vi "Main UI.vi"() -> ()   [LabVIEW 2015, in "Application.lvclass"]
uses:
  Application.lvclass
  EXECUTION_UI_STATE_TYPEDEF.ctl
  Project.lvclass
panel:
  in  "StopBtn":bool
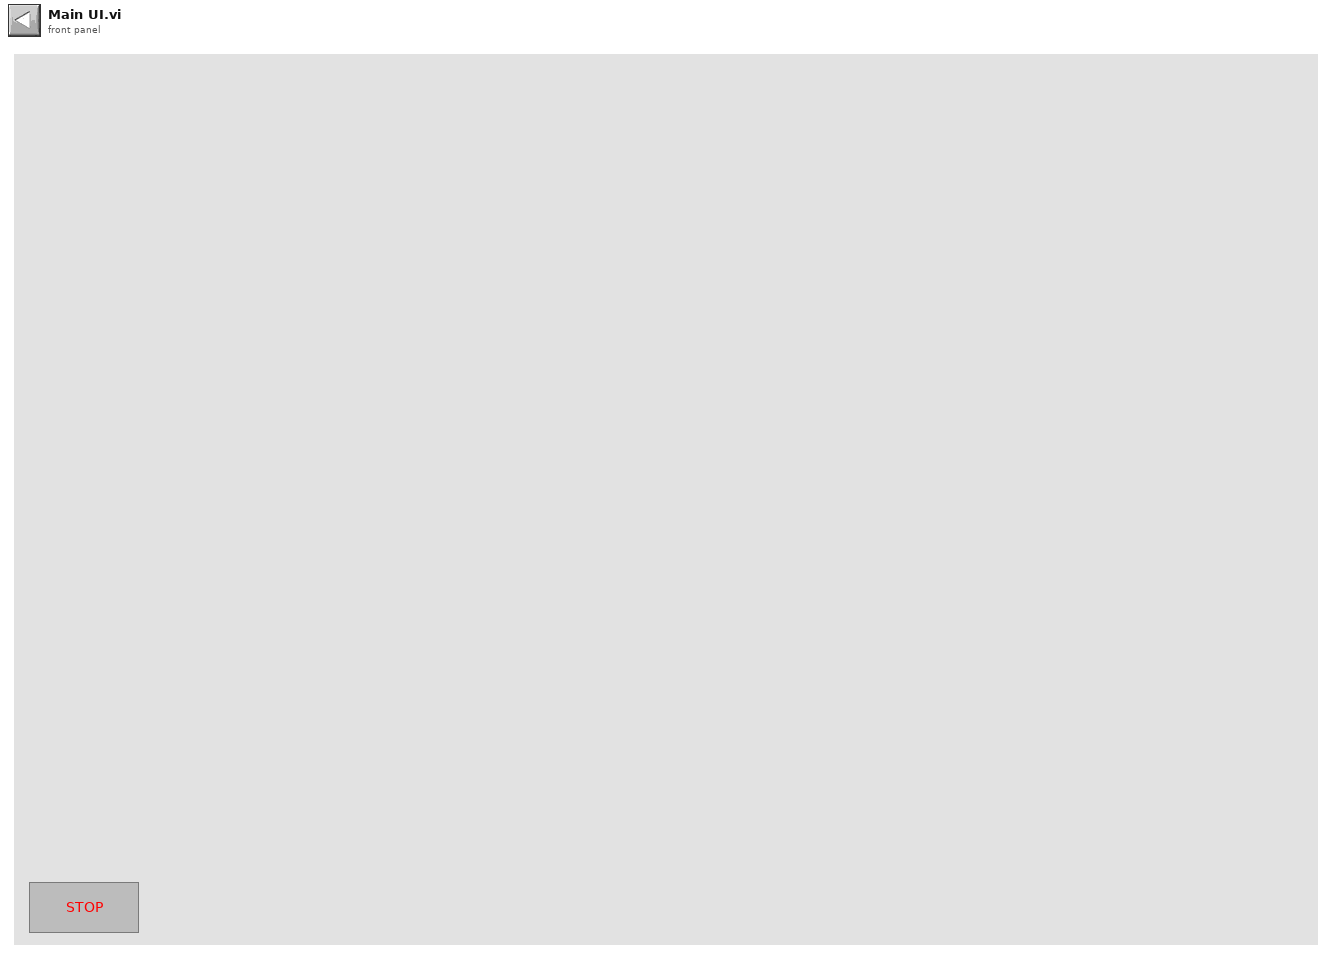
[diagram p1: front panel]
types:
  T1 = typedef "Application.lvclass/EXECUTION_UI_STATE_TYPEDEF.ctl" = enum16{"EXIT", "UI_LOOP", "LOAD_PROJ", "LOG_VIEWER", "PLUGIN_OPTIONS", "APP_OPTIONS", "ABOUT_TESTLITE"}
  T2 = enum32{"Invalid", "Standard", "Closed", "Hidden", "Minimized", "Maximized"}
  T3 = enum32{"invalid app kind", "Development System", "Run Time System", "Student Edition", "Embedded LabVIEW", "Evaluation", "Custom"}
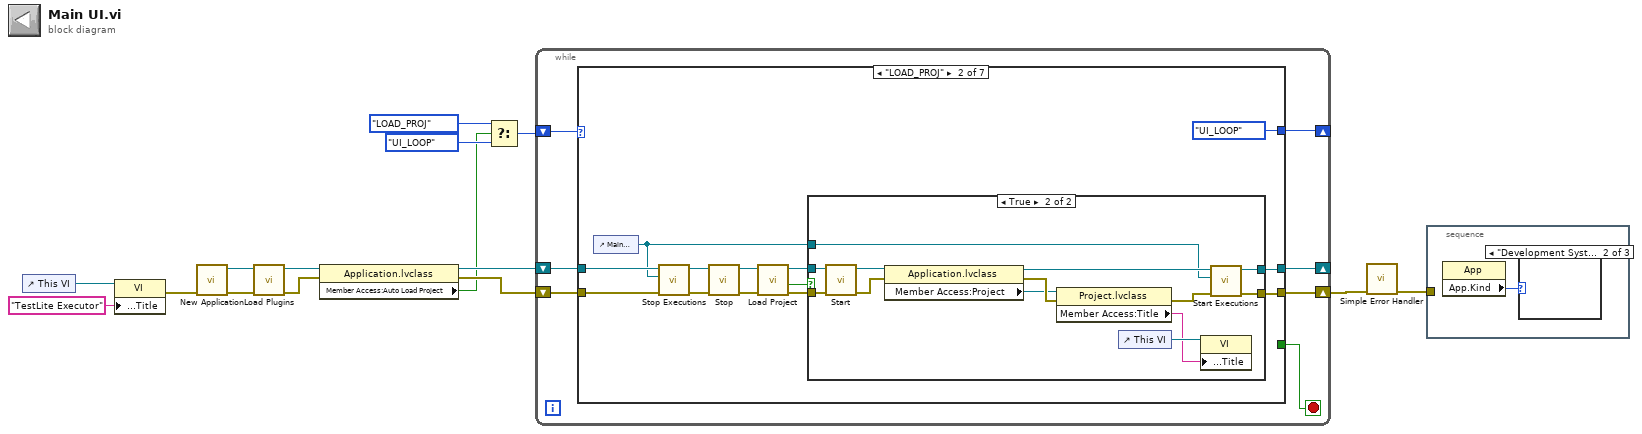
[diagram p0: block diagram]
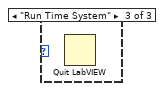
[diagram p3: hidden frame]
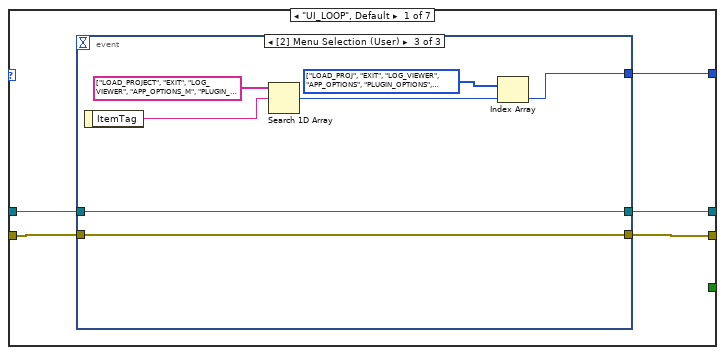
[diagram p4: hidden frame]
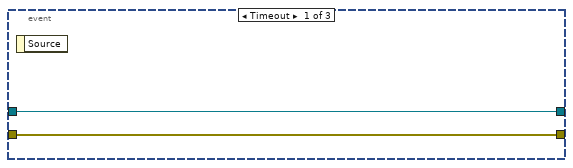
[diagram p5: hidden frame]
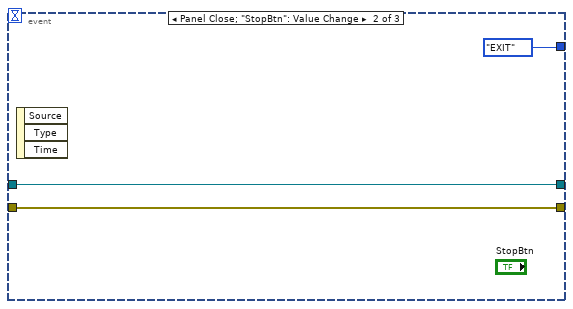
[diagram p6: hidden frame]
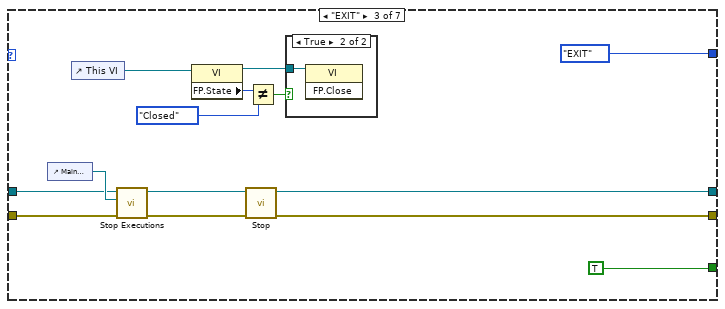
[diagram p8: hidden frame]
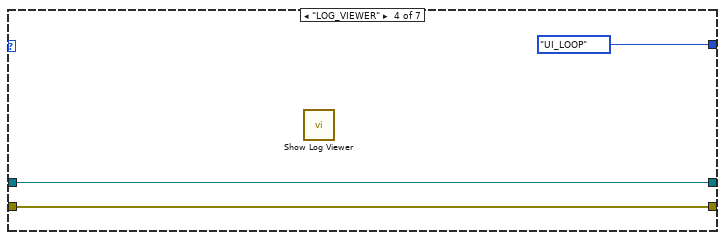
[diagram p10: hidden frame]
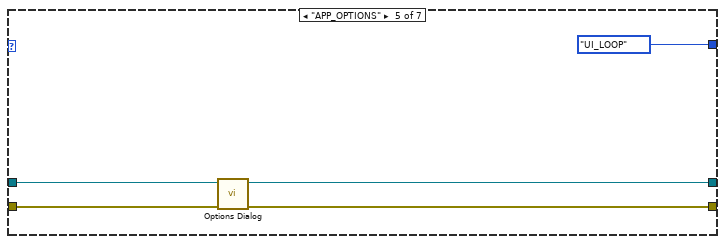
[diagram p11: hidden frame]
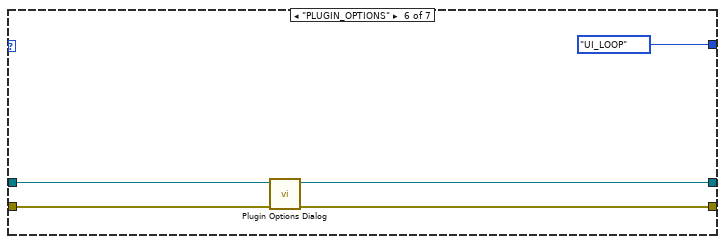
[diagram p12: hidden frame]
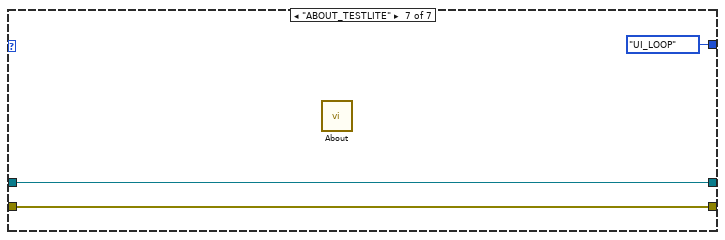
[diagram p13: hidden frame]
diagram:
  n1 = control-ref of="This VI"() -> (w3:refnum<vi>)
  n2 = property class="VI"(reference=w3, "Front Panel.Title"="TestLite Executor" ("Front Panel Window:Title")) -> (error out=w2:errorcluster)  [unwired: 1 in, 1 out]
  n3 = call "New Application.vi"("error in (no error)"=w2) -> ("error out"=w13:errorcluster, "Application"=w14:refnum<data-value>)  [unwired: 9 in]
  n4 = call "Load Plugins.vi"("error in (no error)"=w13, "Application in"=w14) -> ("error out"=w10:errorcluster, "Application out"=w11:refnum<data-value>)  [unwired: 8 in]
  n5 = property class="Application.lvclass"(reference=w11, error in=w10) -> (reference out=w9:refnum<data-value>, error out=w8:errorcluster, "Member Access:Auto Load Project"=w4:bool)
  n6 = Select(t=EXECUTION_UI_STATE_TYPEDEF."LOAD_PROJ", s=w4, f=EXECUTION_UI_STATE_TYPEDEF."UI_LOOP") -> (s? t:f=w5:T1)
  n7 = while {
    shift-right: [w19] -> _
    shift-left: w9 -> [w21]
    shift-right: [w18] -> w12
    shift-left: w8 -> [w20]
    shift-right: [w16] -> _
    shift-left: w5 -> [w22]
    stop <- w17 stop-if-true
    n8 = case shown="\"LOAD_PROJ\"" w22 {
      tunnel: w21 -> [w27 w47 w77 w84 w90 w95 w98]
      tunnel: w20 -> [w26 w46 w78 w83 w89 w94 w97]
      tunnel: [w25 w49 w71 w84 w88 w93 w98] -> w19
      tunnel: [w24 w48 w70 w83 w87 w92 w97] -> w18
      tunnel: [_ _ TRUE _ _ _ _] -> w17
      tunnel: [w23 EXECUTION_UI_STATE_TYPEDEF."UI_LOOP" EXECUTION_UI_STATE_TYPEDEF."EXIT" EXECUTION_UI_STATE_TYPEDEF."UI_LOOP" EXECUTION_UI_STATE_TYPEDEF."UI_LOOP" EXECUTION_UI_STATE_TYPEDEF."UI_LOOP" EXECUTION_UI_STATE_TYPEDEF."UI_LOOP"] -> w16
      frame "UI_LOOP", Default {
        n9 = event shown="[2] Menu Selection (User)" {
          selector: _ -> [_ _ _]
          dyn-events: _ -> [_ _ _]
          timeout: _ -> [_ _ _]
          tunnel: w27 -> [w29 w32 w39]
          tunnel: [w29 w32 w39] -> w25
          tunnel: w26 -> [w28 w31 w38]
          tunnel: [w28 w31 w38] -> w24
          tunnel: [_ EXECUTION_UI_STATE_TYPEDEF."EXIT" w35] -> w23
          event Timeout {
            n10 = event-data() -> ()  [unwired: 1 in, 1 out]
          }
          event Panel Close; "StopBtn": Value Change {
            n11 = event-data() -> ()  [unwired: 1 in, 3 out]
          }
          event Menu Selection (User) {
            w33 = T1[] [enum."LOAD_PROJ", enum."EXIT", enum."LOG_VIEWER", enum."APP_OPTIONS", enum."PLUGIN_OPTIONS", enum."ABOUT_TESTLITE"] items=["EXIT", "UI_LOOP", "LOAD_PROJ", "LOG_VIEWER", "PLUGIN_OPTIONS", "APP_OPTIONS", "ABOUT_TESTLITE"]
            n12 = event-data() -> ("ItemTag"=w37:string)  [unwired: 1 in]
            n13 = Search 1D Array(1D array=string[] ["LOAD_PROJECT", "EXIT", "LOG_VIEWER", "APP_OPTIONS_M", "PLUGIN_OPTIONS", "ABOUT_TESTLITE"], element=w37) -> (index of element=w36:i32)  [unwired: 1 in]
            n14 = Index Array(array=w33, index=w36) -> (element=w35:T1)
          }
        }
      }
      frame "LOAD_PROJ" {
        n15 = control-ref of="Main Continer"() -> (w45:refnum<vi>)
        n16 = call "Stop Executions.vi"("error in (no error)"=w46, "Main Continer"=w45, "Application in"=w47) -> ("error out"=w40:errorcluster, "Application out"=w43:refnum<data-value>)  [unwired: 7 in]
        n17 = call "Stop.vi"("error in (no error)"=w40, "Application in"=w43) -> ("error out"=w41:errorcluster, "Application out"=w42:refnum<data-value>)  [unwired: 8 in]
        n18 = call "Load Project.vi"("error in (no error)"=w41, "Application in"=w42) -> ("error out"=w51:errorcluster, "Succeed"=w44:bool, "Application out"=w50:refnum<data-value>)  [unwired: 7 in]
        n19 = case shown="True" w44 {
          tunnel: w51 -> [w53 w65]
          tunnel: w50 -> [w54 w64]
          tunnel: [w54 w57] -> w49
          tunnel: [w53 w56] -> w48
          tunnel: w45 -> [_ w55]
          frame False {
          }
          frame True {
            n20 = call "Start.vi"("error in (no error)"=w65, "Application in"=w64) -> ("error out"=w67:errorcluster, "Application out"=w66:refnum<data-value>)  [unwired: 8 in]
            n21 = property class="Application.lvclass"(reference=w66, error in=w67) -> (reference out=w63:refnum<data-value>, error out=w61:errorcluster, "Member Access:Project"=w59:refnum<class "Project.lvclass">)
            n22 = property class="Project.lvclass"(reference=w59, error in=w61) -> (error out=w62:errorcluster, "Member Access:Title"=w58:string)  [unwired: 1 out]
            n23 = control-ref of="This VI"() -> (w60:refnum<vi>)
            n24 = property class="VI"(reference=w60, "Front Panel.Title"=w58) -> ()  [unwired: 1 in, 2 out]
            n25 = call "Start Executions.vi"("error in (no error)"=w62, "Main Continer"=w55, "Application in"=w63) -> ("error out"=w56:errorcluster, "Application out"=w57:refnum<data-value>)  [unwired: 7 in]
          }
        }
      }
      frame "EXIT" {
        n26 = control-ref of="Main Continer"() -> (w81:refnum<vi>)
        n27 = control-ref of="This VI"() -> (w72:refnum<vi>)
        n28 = call "Stop Executions.vi"("error in (no error)"=w78, "Main Continer"=w81, "Application in"=w77) -> ("error out"=w80:errorcluster, "Application out"=w79:refnum<data-value>)  [unwired: 7 in]
        n29 = property class="VI"(reference=w72) -> (reference out=w76:refnum<vi>, "FP.State"=w73:T2)  [unwired: 1 in, 1 out]
        n30 = call "Stop.vi"("error in (no error)"=w80, "Application in"=w79) -> ("error out"=w70:errorcluster, "Application out"=w71:refnum<data-value>)  [unwired: 8 in]
        n31 = Not Equal?(x=w73, y=T2."Closed") -> (x != y?=w75:bool)
        n32 = case shown="True" w75 {
          tunnel: w76 -> [_ w82]
          frame False {
          }
          frame True {
            n33 = invoke class="VI" method="FP.Close"(reference=w82) -> ()  [unwired: 2 in, 3 out]
          }
        }
      }
      frame "LOG_VIEWER" {
        n34 = call "Show Log Viewer.vi"() -> ()  [unwired: 12 in]
      }
      frame "APP_OPTIONS" {
        n35 = call "Options Dialog.vi"("error in (no error)"=w89, "Application in"=w90) -> ("error out"=w87:errorcluster, "Application out"=w88:refnum<data-value>)  [unwired: 8 in]
      }
      frame "PLUGIN_OPTIONS" {
        n36 = call "Plugin Options Dialog.vi"("error in (no error)"=w94, "Application in"=w95) -> ("error out"=w92:errorcluster, "Application out"=w93:refnum<data-value>)  [unwired: 8 in]
      }
      frame "ABOUT_TESTLITE" {
        n37 = call "About.vi"() -> ()  [unwired: 12 in]
      }
    }
  }
  n38 = call <vilib>:"Simple Error Handler.vi"("error in (no error)"=w12) -> ("error out"=w15:errorcluster)  [unwired: 4 in, 4 out]
  n39 = stacked-sequence {
    tunnel: w15 -> [_]
    frame #0 {
      n40 = property class="App"() -> ("App.Kind"=w99:T3)  [unwired: 2 in, 2 out]
      n41 = case shown="\"Development System\"" w99 {
        frame "invalid app kind", Default {
        }
        frame "Development System" {
        }
        frame "Run Time System" {
          n42 = Quit LabVIEW() -> ()  [unwired: 1 in]
        }
      }
    }
  }
